vi "array -- hash table -- enum based.vi"(0 "key table":T2[](array[typedef]), 2 "value table":T1[](array[typedef]), 6 "hash action":T3) -> (14 "Key table OUT":T2[](array[typedef]), 16 "value table OUT":T1[](array[typedef]), 17 "torque -- hash value OUT":T1={"time (sec) array"=[], "temperature (K) array"=[], "SRS Vx (V) array"=[], "field (T) array"=[], "filename"="name"}, 18 "index":i32, 19 "found?":bool)   [LabVIEW 2012]
uses:
  hash status control.ctl
  stack action -- control.ctl
  hash action control.ctl
  torque -- hash key.ctl
  torque -- hash value.ctl
panel:
  in  "hash":refnum<vi>
  in  "Enum":enum16{""}(ring)
  out "hash key 2":string
  in  "hash key":string
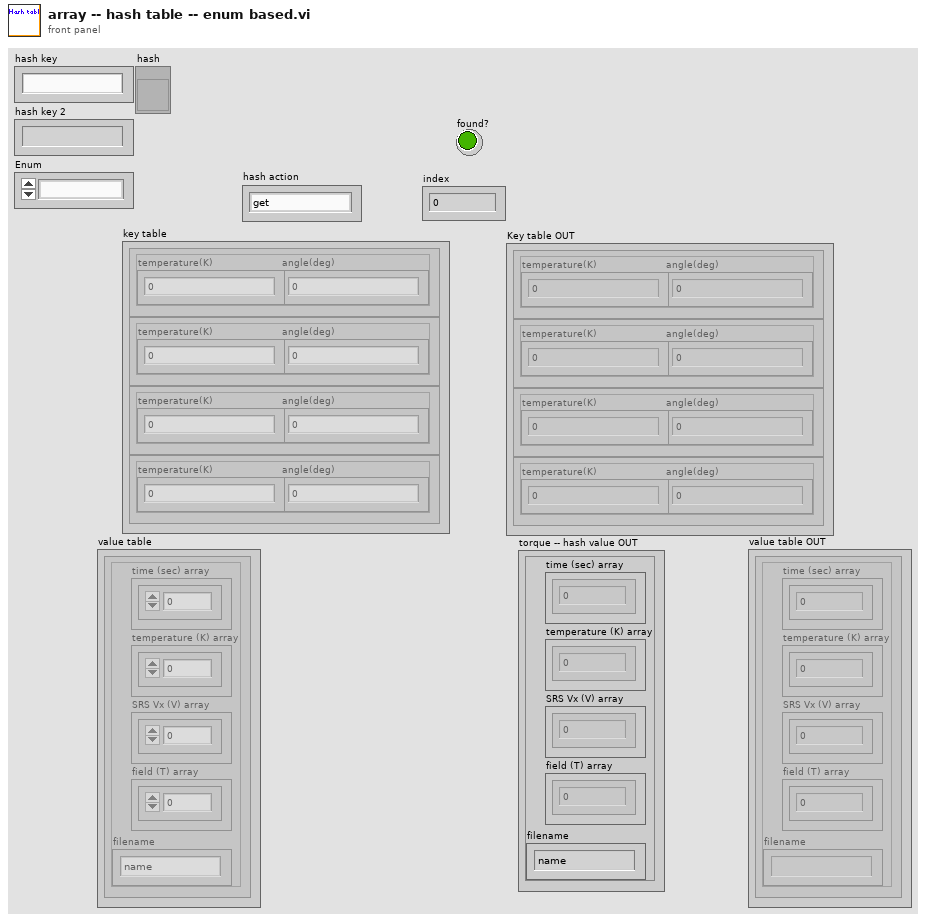
[diagram p1: front panel]
types:
  T1 = typedef "torque -- hash value.ctl" = cluster{"time (sec) array":dbl[], "temperature (K) array":dbl[], "SRS Vx (V) array":dbl[], "field (T) array":dbl[], "filename":string}
  T2 = typedef "torque -- hash key.ctl" = cluster{"temperature(K)":dbl, "angle(deg)":dbl}
  T3 = typedef "hash action control.ctl" = enum16{"get", "new", "--void", "delete", "delete all", "set", "--delete if exists", "--create if not there", "list keys"}
  T4 = typedef "stack action -- control.ctl" = enum16{"push", "pop", "check", "init"}
  T5 = typedef "hash status control.ctl" = enum16{"exists", "does not exists"}
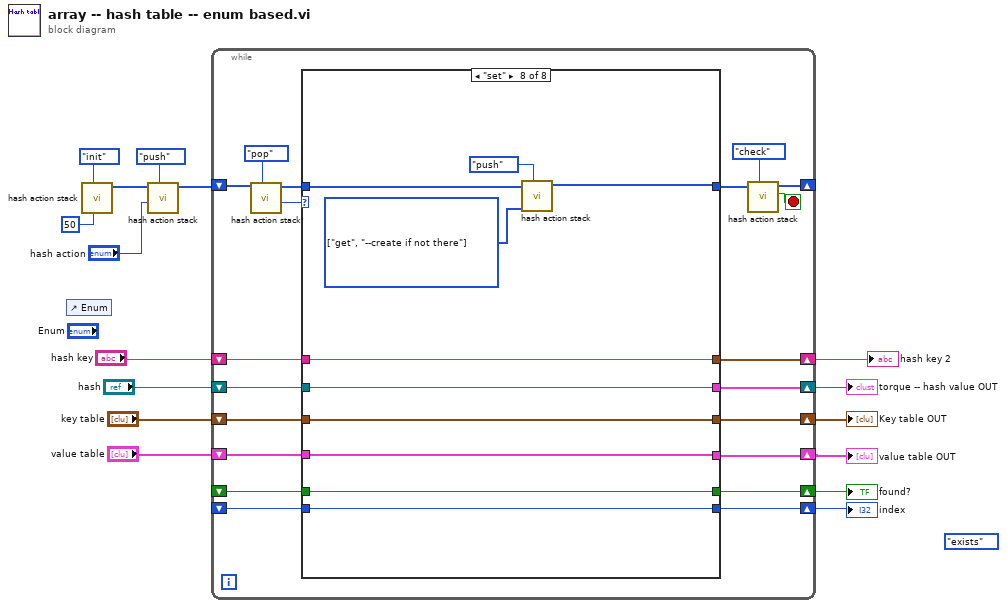
[diagram p0: block diagram]
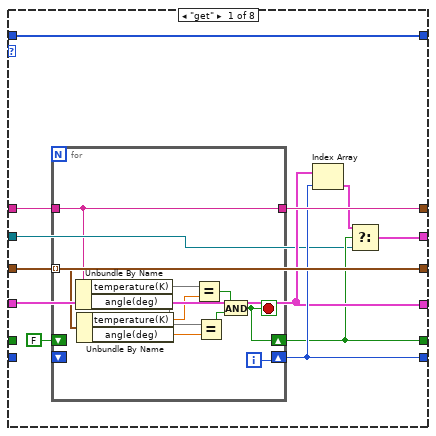
[diagram p2: hidden frame]
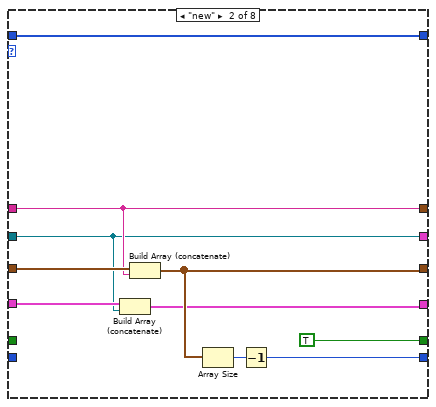
[diagram p3: hidden frame]
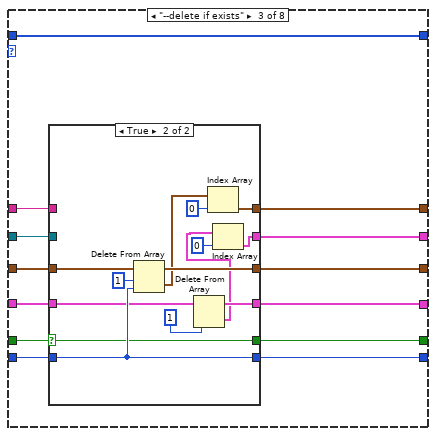
[diagram p4: hidden frame]
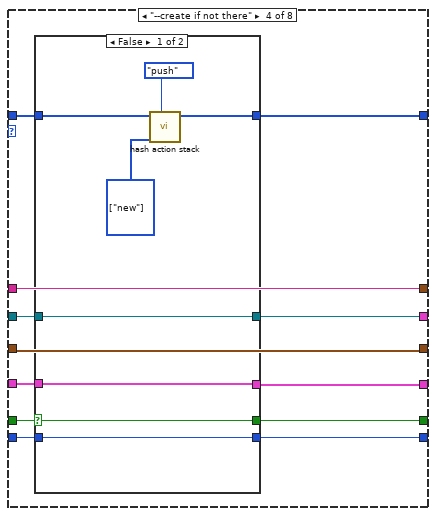
[diagram p6: hidden frame]
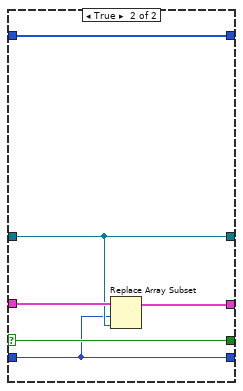
[diagram p7: hidden frame]
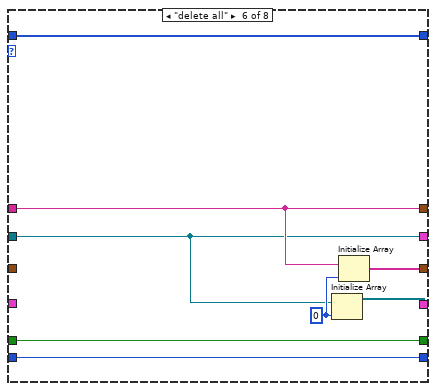
[diagram p9: hidden frame]
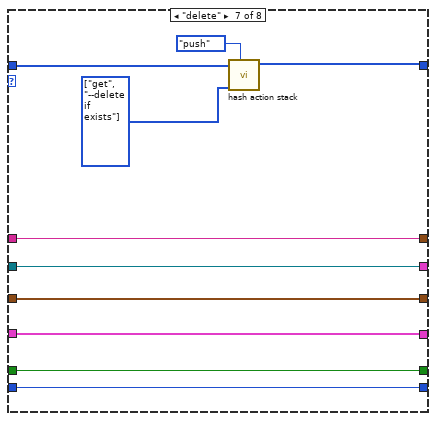
[diagram p10: hidden frame]
diagram:
  (unwired) hash_status_control."exists" ("hash status")
  n1 = control-ref of="Enum"() -> ()  [unwired: 1 out]
  n2 = call "hash action stack.vi"("init size"=50 ("dimension size"), "stack action"=stack_action_--_control."init") -> ("command stack out"=w12:T3[])  [unwired: 7 in, 2 out]
  n3 = call "hash action stack.vi"("stack action"=stack_action_--_control."push", "hash action"="hash action", "command stack"=w12) -> ("command stack out"=w14:T3[])  [unwired: 6 in, 2 out]
  n4 = while {
    shift-right: [w30] -> _
    shift-left: w14 -> [w29]
    shift-right: [w27] -> w9
    shift-left: _ -> [w21]
    shift-right: [w28] -> w10
    shift-left: _ -> [w22]
    shift-right: [w26] -> w8
    shift-left: "key table" -> [w23]
    shift-right: [w25] -> w2
    shift-left: "hash key" -> [w24]
    shift-right: [w20] -> w6
    shift-left: "hash" -> [w18]
    shift-right: [w17] -> w5
    shift-left: "value table" -> [w19]
    stop <- w31 stop-if-true
    n5 = call "hash action stack.vi"("stack action"=stack_action_--_control."pop", "command stack"=w29) -> ("cursor window action out"=w32:T3, "command stack out"=w35:T3[])  [unwired: 7 in, 1 out]
    n6 = case shown="\"set\"" w32 {
      tunnel: w35 -> [w47 w67 w80 w106 w133 w141 w145 w153]
      tunnel: [w47 w67 w80 w105 w133 w141 w144 w152] -> w33
      tunnel: w23 -> [w43 w66 w79 w107 w131 _ w150 w160]
      tunnel: w24 -> [w46 w65 w72 w112 w132 w137 w151 w161]
      tunnel: [w40 TRUE w74 w108 w130 w140 w149 w159] -> w28
      tunnel: [w42 w62 w75 w109 w129 w139 w148 w158] -> w27
      tunnel: [w43 w64 w78 w107 w131 w136 w150 w160] -> w26
      tunnel: [w44 w65 w73 w112 w132 w137 w151 w161] -> w25
      tunnel: w22 -> [_ _ w76 w110 w130 w140 w149 w159]
      tunnel: w21 -> [_ _ w77 w111 w129 w139 w148 w158]
      tunnel: [w38 w59 w71 w101 w128 w135 w143 w155] -> w20
      tunnel: w18 -> [w37 w59 w70 w102 w128 w135 w143 w155]
      tunnel: w19 -> [w41 w60 w68 w104 w127 _ w142 w154]
      tunnel: [w41 w58 w69 w103 w127 w134 w142 w154] -> w17
      frame "get" {
        n7 = for {
          tunnel: w43 -> [w49] mode=indexing
          tunnel: w46 -> [w48]
          shift-right: [w51] -> w40
          shift-left: FALSE -> [_]
          shift-right: [w50] -> w42
          shift-left: _ -> [_]
          tunnel: [w48] -> w44
          i -> [w50]
          stop <- w51 stop-if-true
          n8 = Unbundle By Name(w48) -> ("temperature(K)"=w56, "angle(deg)"=w55)
          n9 = Unbundle By Name(w49) -> ("temperature(K)"=w57:dbl, "angle(deg)"=w54:dbl)
          n10 = Equal?(x=w56, y=w57) -> (x = y?=w53:bool)
          n11 = Equal?(x=w55, y=w54) -> (x = y?=w52:bool)
          n12 = And(x=w53, y=w52) -> (x .and. y?=w51:bool)
        }
        n13 = Index Array(array=w41, index=w42) -> (element=w39:T1)
        n14 = Select(t=w39, s=w40, f=w37) -> (s? t:f=w38:T1)
      }
      frame "new" {
        n15 = Build Array (concatenate)(w60, w59) -> (w58:T1[])
        n16 = Build Array (concatenate)(w66, w65) -> (w64:T2[])
        n17 = Array Size(array=w64) -> (size(s)=w63:i32)
        n18 = Decrement(x=w63) -> (x-1=w62:i32)
      }
      frame "--delete if exists" {
        n19 = case shown="True" w76 {
          selector: w76 -> [w85 w96]
          tunnel: w79 -> [w86 w100]
          tunnel: [w86 w99] -> w78
          tunnel: w77 -> [w84 w97]
          tunnel: [w84 w97] -> w75
          tunnel: [w85 w96] -> w74
          tunnel: [w83 w93] -> w73
          tunnel: w72 -> [w83 _]
          tunnel: [w82 w88] -> w71
          tunnel: w70 -> [w82 _]
          tunnel: [w81 w91] -> w69
          tunnel: w68 -> [w81 w90]
          frame False {
          }
          frame True {
            n20 = Delete From Array(array=w100, length=1, index=w97) -> (deleted portion=w95:T2[], array with subset deleted=w99:T2[])
            n21 = Delete From Array(array=w90, length=1) -> (deleted portion=w87:T1[], array with subset deleted=w91:T1[])  [unwired: 1 in]
            n22 = Index Array(array=w95, index=0) -> (element=w93:T2)
            n23 = Index Array(array=w87, index=0) -> (element=w88:T1)
          }
        }
      }
      frame "--create if not there" {
        n24 = case shown="False" w110 {
          selector: w110 -> [w119 w126]
          tunnel: w111 -> [w120 w121]
          tunnel: [w120 w121] -> w109
          tunnel: [w119 w126] -> w108
          tunnel: w106 -> [w117 w125]
          tunnel: [w116 w125] -> w105
          tunnel: w104 -> [w114 w124]
          tunnel: [w114 w123] -> w103
          tunnel: w102 -> [w115 w122]
          tunnel: [w115 w122] -> w101
          frame False {
            w113 = T3[] [enum."new"] items=["get", "new", "--void", "delete", "delete all", "set", "--delete if exists", "--create if not there", "list keys"] ("hash action list")
            n25 = call "hash action stack.vi"("stack action"=stack_action_--_control."push", "hash action list"=w113, "command stack"=w117) -> ("command stack out"=w116:T3[])  [unwired: 6 in, 2 out]
          }
          frame True {
            n26 = Replace Array Subset(array=w124, new element=w122, index=w121) -> (w123:T1[])
          }
        }
      }
      frame "--void", Default {
      }
      frame "delete all" {
        w138 = 0 ("dimension size")
        n27 = Initialize Array(w135, w138) -> (w134:refnum<vi>[])
        n28 = Initialize Array(w137, w138) -> (w136:string[])
      }
      frame "delete" {
        w146 = T3[] [enum."get", enum."--delete if exists"] items=["get", "new", "--void", "delete", "delete all", "set", "--delete if exists", "--create if not there", "list keys"] ("hash action list")
        n29 = call "hash action stack.vi"("stack action"=stack_action_--_control."push", "hash action list"=w146, "command stack"=w145) -> ("command stack out"=w144:T3[])  [unwired: 6 in, 2 out]
      }
      frame "set" {
        w156 = T3[] [enum."get", enum."--create if not there"] items=["get", "new", "--void", "delete", "delete all", "set", "--delete if exists", "--create if not there", "list keys"] ("hash action list")
        n30 = call "hash action stack.vi"("stack action"=stack_action_--_control."push", "hash action list"=w156, "command stack"=w153) -> ("command stack out"=w152:T3[])  [unwired: 6 in, 2 out]
      }
    }
    n31 = call "hash action stack.vi"("stack action"=stack_action_--_control."check", "command stack"=w33) -> ("stack is empty ?"=w31:bool, "command stack out"=w30:T3[])  [unwired: 7 in, 1 out]
  }
  "found?" <- w10
  "index" <- w9
  "Key table OUT" <- w8
  "torque -- hash value OUT" <- w6
  "value table OUT" <- w5
  "hash key 2" <- w2
